vi "Read Waveforms.vi"   [LabVIEW 2010, in "Agilent 2000 3000 X-Series.lvlib"]
doc: "Reads waveforms data."
uses:
  <instrlib>/Agilent 2000 3000 X-Series/Agilent 2000 3000 X-Series.lvlib
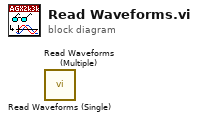
[diagram p0: block diagram]
diagram:
  n1 = call <instrlib>:"Read Waveforms (Single).vi"() -> ()  [unwired: 9 in, 3 out]
  n2 = call <instrlib>:"Read Waveforms (Multiple).vi"() -> ()  [unwired: 9 in, 3 out]
